vi "Generate Chessboard Image Data.vi"   [LabVIEW 2020, in "feature_detection.lvlib"]
doc: "Generate a chessboard for use with the Find Chessboard Corners Function and Camera Calibration."
uses:
  feature_detection.lvlib
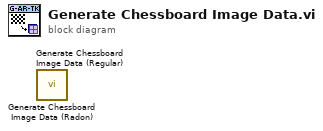
[diagram p0: block diagram]
diagram:
  n1 = call "Generate Chessboard Image Data (Radon).vi"() -> ()  [unwired: 10 in, 2 out]
  n2 = call "Generate Chessboard Image Data (Regular).vi"() -> ()  [unwired: 10 in, 2 out]
